vi "LoadMonitor.vi"(1 "error out":errorcluster, 2 "hostname":string) -> (0 "error IO":errorcluster)   [LabVIEW 2018, in "feGEM DataPacker.lvlib"]
uses:
  feGEM DataPacker.lvlib
  SendStuff/SlowLogger.lvclass
  SendStuff/SlowLogger.lvclass/SlowLogger.ctl
  SendStuff/SlowLogger_LogThisSlowly.vi/f93abad2-5217-430f-97d3-b2f2641e9ea3.vi
  SendStuff/SlowLogger_LogThisSlowly.vi/f93abad2-5217-430f-97d3-b2f2641e9ea3.vi/8e3691a2-e3c2-4584-a4da-cc476d1f3f0f.vi
  <resource>/objmgr/nisysapi.rc
  <resource>/objmgr/motionsysapi.rc
panel:
  out "CPUMEM LOAD (%)":sgl[](array[numeric])
  in  "stop":bool
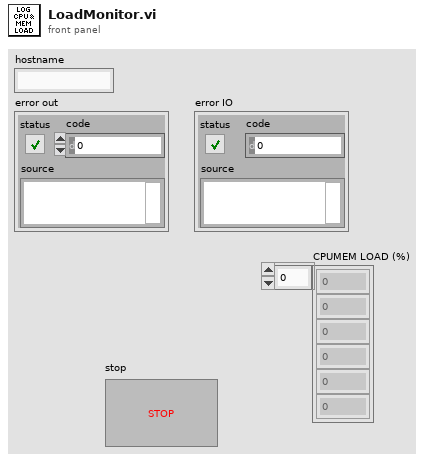
[diagram p1: front panel]
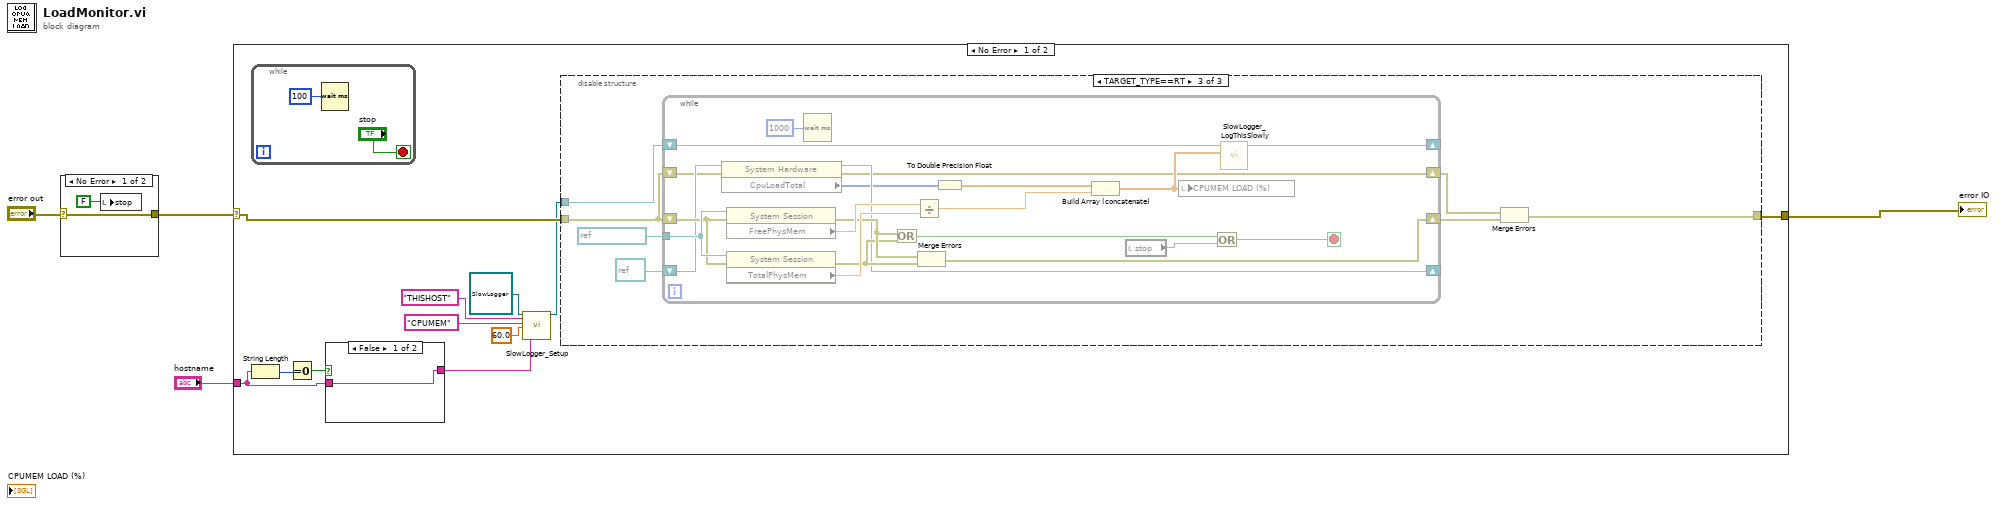
[diagram p0: block diagram]
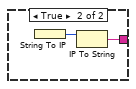
[diagram p3: hidden frame]
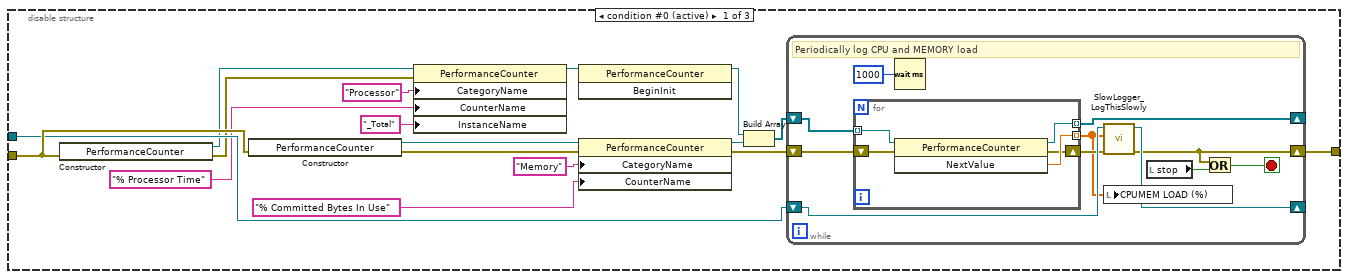
[diagram p4: hidden frame]
diagram:
  n1 = case shown="No Error" "error out" {
    selector: "error out" -> [w5 w7]
    tunnel: [w5 w7] -> w1
    frame No Error {
      n2 = local write "stop"(FALSE) -> ()
    }
    frame Error {
    }
  }
  n3 = case shown="No Error" w1 {
    selector: w1 -> [w17 w85]
    tunnel: "hostname" -> [w14 _]
    tunnel: [w18 w85] -> w3
    frame No Error {
      n4 = while {
        stop <- "stop" stop-if-true
        n5 = Wait (ms)(milliseconds to wait=u32 100) -> ()  [unwired: 1 out]
      }
      n6 = String Length(string=w14) -> (length=w16:i32)
      n7 = Equal To 0?(x=w16) -> (x = 0?=w15:bool)
      n8 = case shown="False" w15 {
        tunnel: w14 -> [w21 _]
        tunnel: [w21 w22] -> w13
        frame False {
        }
        frame True {
          n9 = String To IP() -> (0:w23:u32)  [unwired: 1 in]
          n10 = IP To String(2:w23) -> (0:w22:string)  [unwired: 1 in]
        }
      }
      n11 = call "SlowLogger_Setup.vi"("SlowLogger in"=refnum<class "SlowLogger.lvclass"> refnum ("SlowLogger.lvclass"), "Category"="THISHOST", "Variable Name"="CPUMEM", "Max Log Speed [Delta Time] (seconds)"=60.0, "Equipment Description (32 chars)"=w13) -> ("SlowLogger out"=w8:refnum<class "SlowLogger.lvclass">)  [unwired: 13 in, 1 out]
      n12 = disable-structure shown="TARGET_TYPE==RT" {
        disable-tunnel: w17 -> [w36 _ w60]
        disable-tunnel: [w32 _ w57] -> w18
        disable-tunnel: w8 -> [w35 _ w59]
        frame condition #0 (active) {
          n13 = constructor class="PerformanceCounter" ("Constructor Node")(error in=w36) -> (reference out=w29:refnum<k24>, error out=w28:errorcluster)  [unwired: 2 in, 1 out]
          n14 = constructor class="PerformanceCounter" ("Constructor Node")(error in=w36) -> (reference out=w39:refnum<k24>, error out=w40:errorcluster)  [unwired: 2 in, 1 out]
          n15 = property on="Property Node" class="PerformanceCounter"(reference=w29, error in=w28, "CategoryName"="Processor", "CounterName"="% Processor Time", "InstanceName"="_Total") -> (reference out=w30:refnum<k24>)  [unwired: 1 out]
          n16 = invoke class="PerformanceCounter" method="BeginInit"(reference=w30) -> (reference out=w24:refnum<k24>)  [unwired: 2 in, 2 out]
          n17 = property on="Property Node" class="PerformanceCounter"(reference=w39, error in=w40, "CategoryName"="Memory", "CounterName"="% Committed Bytes In Use") -> (reference out=w34:refnum<k24>, error out=w31:errorcluster)
          n18 = Build Array(w24, w34) -> (w33:refnum<k24>[])
          n19 = while {
            shift-right: [w42] -> w32
            shift-left: w31 -> [w45]
            shift-right: [w48] -> _
            shift-left: w35 -> [w49]
            shift-right: [w41] -> _
            shift-left: w33 -> [w46]
            stop <- w51 stop-if-true
            # "Periodically log CPU and MEMORY load"
            n20 = for {
              tunnel: w46 -> [w56] mode=indexing
              tunnel: [w55] -> w43 mode=indexing
              shift-right: [w53] -> w44
              shift-left: w45 -> [w54]
              tunnel: [w52] -> w41 mode=indexing
              n21 = invoke on="Invoke Node" class="PerformanceCounter" method="NextValue"(reference=w56, error in=w54) -> (reference out=w52:refnum<k24>, error out=w53:errorcluster, "NextValue"=w55:sgl)  [unwired: 1 in]
            }
            n22 = Wait (ms)(milliseconds to wait=u32 1000) -> ()  [unwired: 1 out]
            n23 = call "SlowLogger_LogThisSlowly.vi"("error in (no error)"=w44, "Array"=w43, "SlowLogger in"=w49) -> ("error out"=w42:errorcluster, "SlowLogger out"=w48:refnum<class "SlowLogger.lvclass">)  [unwired: 5 in, 2 out]
            n24 = local write "CPUMEM LOAD (%)"(w43) -> ()
            n25 = local read "stop"() -> (w50:bool)
            n26 = Or(x=w42, y=w50) -> (x .or. y?=w51:bool)
          }
        }
        frame condition #1 {
        }
        frame condition #2 {
          n27 = while {
            tunnel: refnum<k21> "localhost" ("System Configuration") -> [w82]
            shift-right: [w70] -> w61
            shift-left: w60 -> [w81]
            shift-right: [w64] -> w62
            shift-left: w60 -> [w65]
            shift-right: [w76] -> _
            shift-left: w59 -> [w77]
            shift-right: [w68] -> _
            shift-left: refnum<k20> refnum ("System Hardware") -> [w69]
            stop <- w73 stop-if-true
            n28 = property class="System Hardware"(reference=w69, error in=w65) -> (reference out=w68:refnum<k20>, error out=w64:errorcluster, "CpuLoadTotal"=w67:u32[])
            n29 = property class="System Session"(reference=w82, error in=w81) -> (error out=w72:errorcluster, "FreePhysMem"=w83:dbl)  [unwired: 1 out]
            n30 = property class="System Session"(reference=w82, error in=w81) -> (error out=w71:errorcluster, "TotalPhysMem"=w84:dbl)  [unwired: 1 out]
            n31 = Wait (ms)(milliseconds to wait=u32 1000) -> ()  [unwired: 1 out]
            n32 = Or(x=w72, y=w71) -> (x .or. y?=w80:bool)
            n33 = Divide(x=w83, y=w84) -> (x/y=w78:dbl)
            n34 = Merge Errors(w72, w71) -> (w70:errorcluster)
            n35 = To Double Precision Float(number=w67) -> (double precision float=w66:dbl[])
            n36 = Build Array (concatenate)(w66, w78) -> (w74:dbl[])
            n37 = local read "stop"() -> (w79:bool)
            n38 = local write "CPUMEM LOAD (%)"(w74) -> ()
            n39 = Or(x=w80, y=w79) -> (x .or. y?=w73:bool)
            n40 = call "SlowLogger_LogThisSlowly.vi"("Array"=w74, "SlowLogger in"=w77) -> ("SlowLogger out"=w76:refnum<class "SlowLogger.lvclass">)  [unwired: 6 in, 3 out]
          }
          n41 = Merge Errors(w62, w61) -> (w57:errorcluster)
        }
      }
    }
    frame Error {
    }
  }
  "error IO" <- w3
